vi "checkCouplingAndImpedance.vi"(10 "Impedance2":T1, 11 "IVI Refnum in":refnum<k15>) -> (2 "x .or. y?":bool, 3 "IVI Refnum out":refnum<k15>)   [LabVIEW 2011]
uses:
  impedance_Enum_TypDEf.ctl
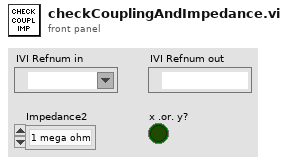
[diagram p1: front panel]
types:
  T1 = typedef "impedance_Enum_TypDEf.ctl" = enum16{"1 mega ohm", "<NA>", "50 ohms"}
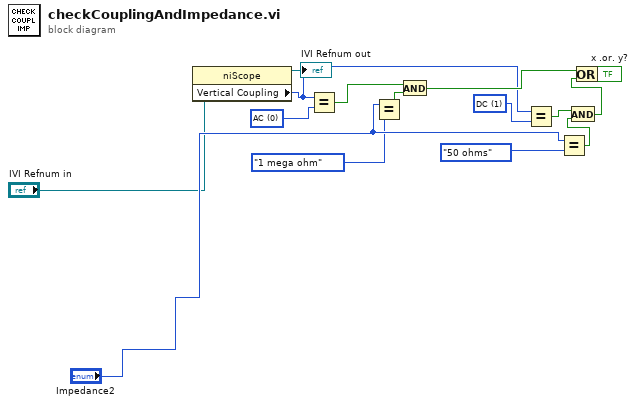
[diagram p0: block diagram]
diagram:
  w5 = 1 items=["AC", "DC", "Ground"] ("Vertical:Vertical Coupling")
  w2 = 0 items=["AC", "DC", "Ground"] ("Vertical:Vertical Coupling")
  n1 = property class="niScope"(reference="IVI Refnum in") -> (reference out=→"IVI Refnum out":refnum<k15>, "Vertical Coupling"=w4:i32)  [unwired: 1 in, 1 out]
  n2 = Equal?(x=w4, y=w2) -> (x = y?=w9:bool)
  n3 = Equal?(x="Impedance2", y=impedance_Enum_TypDEf."1 mega ohm" ("output 1")) -> (x = y?=w8:bool)
  n4 = And(x=w9, y=w8) -> (x .and. y?=w13:bool)
  n5 = Equal?(x=w4, y=w5) -> (x = y?=w10:bool)
  n6 = Equal?(x="Impedance2", y=impedance_Enum_TypDEf."50 ohms" ("output 1")) -> (x = y?=w11:bool)
  n7 = And(x=w10, y=w11) -> (x .and. y?=w12:bool)
  n8 = Or(x=w13, y=w12) -> (x .or. y?=→"x .or. y?":bool)
